vi "Get Supported Targets.vi"(8 "error in":errorcluster, 11 "CVT configuration in":refnum<class "CVT configuration.lvclass">) -> (0 "error out":errorcluster, 2 "supported targets":T1[](array[typedef]), 3 "CVT configuration out":refnum<class "CVT configuration.lvclass">)   [LabVIEW 2013, in "CVT configuration.lvclass"]
doc: "Provides an interface for determining the targets supported by a given module configuration/runtime class pairing. This should be overridden by any useful child class."
uses:
  CVT configuration.lvclass
  <vilib>/NI/Tag Bus Module Framework/root configuration/Target Types.ctl
  <vilib>/NI/Tag Bus Module Framework/root configuration/TBM configuration.lvclass
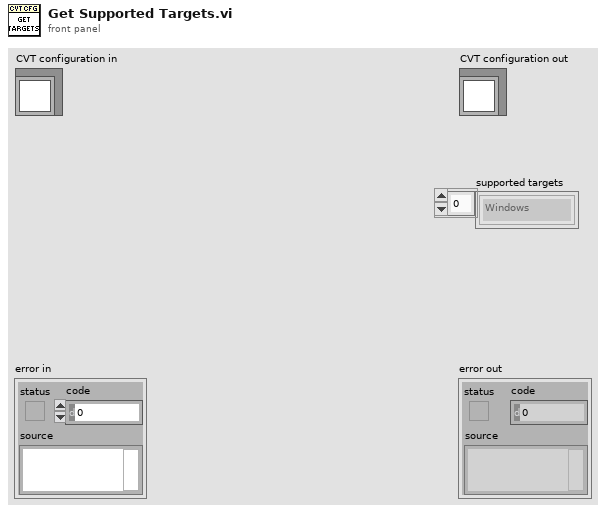
[diagram p1: front panel]
types:
  T1 = typedef "TBM configuration.lvclass/Target Types.ctl" = enum16{"Windows", "Mac", "Linux", "Linux RT", "VxWorks", "Pharlap", "Other"}
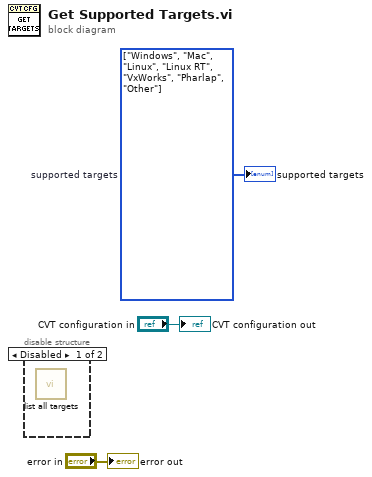
[diagram p0: block diagram]
diagram:
  w1 = T1[] [enum."Windows", enum."Mac", enum."Linux", enum."Linux RT", enum."VxWorks", enum."Pharlap", enum."Other"] items=["Windows", "Mac", "Linux", "Linux RT", "VxWorks", "Pharlap", "Other"]  # supported targets
  n1 = disable-structure shown="Disabled" {
    frame Disabled {
      n2 = call <vilib>:"list all targets.vi"() -> ()  [unwired: 11 in, 1 out]
    }
    frame Enabled {
    }
  }
  "error out" <- "error in"
  "CVT configuration out" <- "CVT configuration in"
  "supported targets" <- w1
